vi "Get 1.3.3 Mutation Chans.vi"() -> (3 "Array":T2(array[cluster]))   [LabVIEW 2020, in "Engine Simulation Toolkit System Explorer.lvlib"]
uses:
  Engine Simulation Toolkit System Explorer.lvlib
  Shared/Channel.ctl
  Shared/Constants and GUIDs.vi
  Shared/Engine Simulation Toolkit Shared.lvlib
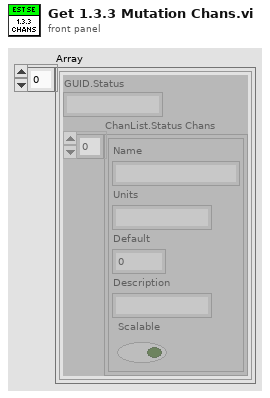
[diagram p1: front panel]
types:
  T1 = typedef "Engine Simulation Toolkit Shared.lvlib/Channel.ctl" = cluster{"Name":string, "Units":string, "Default":dbl, "Description":string, "Scalable":bool}
  T2 = cluster{"GUID.Status":string, "ChanList.Status Chans":T1[]}[]
  T3 = cluster{"GUID.APU Commands":string, "ChanList.APU Commands":T1[]}
  T4 = cluster{"GUID.APU State":string, "ChanList.APU State":T1[]}
  T5 = cluster{"GUID.Analog Replay":string, "ChanList.DataReplayVoltage":T1[]}
  T6 = cluster{"GUID.Faulting":string, "ChanList.DigPtrnFaultingIn":T1[]}
  T7 = cluster{"GUID.Faulting":string, "ChanList.DigPtrnFaultingOut":T1[]}
  T8 = cluster{"GUID.Dir Speed Sensor":string, "ChanList.DirSpeedSensor":T1[]}
  T9 = cluster{"GUID.Event Capture":string, "ChanList.EventCapture":T1[]}
  T10 = cluster{"GUID.Knock Cylinder":string, "ChanList.KnockCylinder":T1[]}
  T11 = cluster{"GUID.Knock Sensor":string, "ChanList.KnockSensor":T1[]}
  T12 = cluster{"GUID.APU State":string, "ChanList.MeasurementStatus":T1[]}
  T13 = cluster{"GUID.Analog Replay":string, "ChanList.Offset":T1[]}
  T14 = cluster{"GUID.Digital Pattern":string, "ChanList.Offset":T1[]}
  T15 = cluster{"GUID.Status":string, "ChanList.Status Chans":T1[]}
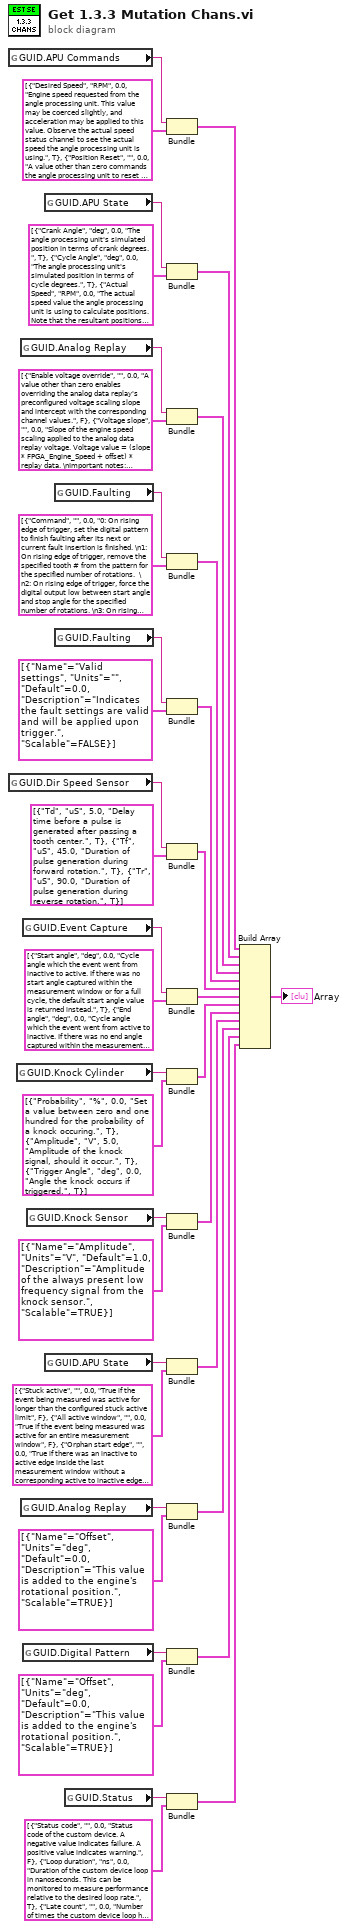
[diagram p0: block diagram]
diagram:
  n1 = global read "Constants and GUIDs.vi" "GUID.APU Commands"() -> (w33:string)
  n2 = global read "Constants and GUIDs.vi" "GUID.Dir Speed Sensor"() -> (w28:string)
  n3 = global read "Constants and GUIDs.vi" "GUID.Knock Cylinder"() -> (w26:string)
  n4 = global read "Constants and GUIDs.vi" "GUID.Analog Replay"() -> (w31:string)
  n5 = global read "Constants and GUIDs.vi" "GUID.Analog Replay"() -> (w23:string)
  n6 = global read "Constants and GUIDs.vi" "GUID.Event Capture"() -> (w27:string)
  n7 = global read "Constants and GUIDs.vi" "GUID.Digital Pattern"() -> (w22:string)
  n8 = global read "Constants and GUIDs.vi" "GUID.Knock Sensor"() -> (w25:string)
  n9 = global read "Constants and GUIDs.vi" "GUID.APU State"() -> (w32:string)
  n10 = global read "Constants and GUIDs.vi" "GUID.APU State"() -> (w24:string)
  n11 = global read "Constants and GUIDs.vi" "GUID.Faulting"() -> (w30:string)
  n12 = global read "Constants and GUIDs.vi" "GUID.Faulting"() -> (w29:string)
  n13 = global read "Constants and GUIDs.vi" "GUID.Status"() -> (w21:string)
  n14 = Bundle("GUID.APU Commands"=w33, "ChanList.APU Commands"=T1[] [{"Name"="Desired Speed", "Units"="RPM", "Default"=0.0, "Description"="Engine speed requested from the angle processing unit. This value may be coerced slightly, and acceleration may be applied to this value. Observe the actual speed status channel to see the actual speed the angle processing unit is using.", "Scalable"=TRUE}, {"Name"="Position Reset", "Units"="", "Default"=0.0, "Description"="A value other than zero commands the angle processing unit to reset to its initial position.\nWARNING: This snaps the angle processing unit position and will cause undefined behavior of output generations for a short time. For example, snapping position could cause a large instantaneous position change resulting in knock simulation generating the knock for several cylinders simultaneously. It is only recommended to reset position when the ECU under test is rebooting.\n", "Scalable"=FALSE}]) -> (w34:T3)  [unwired: 1 in]
  n15 = Bundle("GUID.APU State"=w32, "ChanList.APU State"=T1[] [{"Name"="Crank Angle", "Units"="deg", "Default"=0.0, "Description"="The angle processing unit's simulated position in terms of crank degrees.", "Scalable"=TRUE}, {"Name"="Cycle Angle", "Units"="deg", "Default"=0.0, "Description"="The angle processing unit's simulated position in terms of cycle degrees.", "Scalable"=TRUE}, {"Name"="Actual Speed", "Units"="RPM", "Default"=0.0, "Description"="The actual speed value the angle processing unit is using to calculate positions. Note that the resultant positions will slowly accumulate error as compared to the rotational speed due to numerical representation.", "Scalable"=TRUE}]) -> (w20:T4)  [unwired: 1 in]
  n16 = Bundle("GUID.Analog Replay"=w31, "ChanList.DataReplayVoltage"=T1[] [{"Name"="Enable voltage override", "Units"="", "Default"=0.0, "Description"="A value other than zero enables overriding the analog data replay's preconfigured voltage scaling slope and intercept with the corresponding channel values.", "Scalable"=FALSE}, {"Name"="Voltage slope", "Units"="", "Default"=0.0, "Description"="Slope of the engine speed scaling applied to the analog data replay voltage. Voltage value = (slope * FPGA_Engine_Speed + offset) * replay data. \nImportant notes: Replay data is always normalized to full scale range of the analog output DAC. FPGA_Engine_Speed is equal to RPM * (1/60) * (1/40M) * 2^16.", "Scalable"=TRUE}, {"Name"="Voltage intercept", "Units"="", "Default"=0.0, "Description"="Offset of the engine speed scaling applied to the analog data replay voltage. Voltage value = (slope * FPGA_Engine_Speed + offset) * replay data. \nImportant notes: Replay data is always normalized to full scale range of the analog output DAC. FPGA_Engine_Speed is equal to RPM * (1/60) * (1/40M) * 2^16.", "Scalable"=TRUE}]) -> (w19:T5)  [unwired: 1 in]
  n17 = Bundle("GUID.Faulting"=w30, "ChanList.DigPtrnFaultingIn"=T1[] [{"Name"="Command", "Units"="", "Default"=0.0, "Description"="0: On rising edge of trigger, set the digital pattern to finish faulting after its next or current fault insertion is finished. \n1: On rising edge of trigger, remove the specified tooth # from the pattern for the specified number of rotations.  \n2: On rising edge of trigger, force the digital output low between start angle and stop angle for the specified number of rotations. \n3: On rising edge of trigger, force the digital output high between start angle and stop angle for the specified number of rotations.", "Scalable"=FALSE}, {"Name"="Trigger", "Units"="", "Default"=0.0, "Description"="Ignored if valid settings is false.", "Scalable"=FALSE}, {"Name"="Rotations", "Units"="", "Default"=0.0, "Description"="Up to 16. 0 means indefinitely until faulting is commanded to finish.", "Scalable"=FALSE}, {"Name"="Start angle", "Units"="deg", "Default"=0.0, "Description"="Rotational position to begin faulting.", "Scalable"=TRUE}, {"Name"="Stop angle", "Units"="deg", "Default"=0.0, "Description"="Rotational position to end faulting.", "Scalable"=TRUE}, {"Name"="Tooth to remove", "Units"="", "Default"=0.0, "Description"="Tooth number of the pattern to remove during faulting. Teeth are 1 indexed from the begining of the rotation (crank or cycle) to the end.", "Scalable"=TRUE}]) -> (w18:T6)  [unwired: 1 in]
  n18 = Bundle("GUID.Faulting"=w29, "ChanList.DigPtrnFaultingOut"=T1[] [{"Name"="Valid settings", "Units"="", "Default"=0.0, "Description"="Indicates the fault settings are valid and will be applied upon trigger.", "Scalable"=FALSE}]) -> (w17:T7)  [unwired: 1 in]
  n19 = Bundle("GUID.Dir Speed Sensor"=w28, "ChanList.DirSpeedSensor"=T1[] [{"Name"="Td", "Units"="uS", "Default"=5.0, "Description"="Delay time before a pulse is generated after passing a tooth center.", "Scalable"=TRUE}, {"Name"="Tf", "Units"="uS", "Default"=45.0, "Description"="Duration of pulse generation during forward rotation.", "Scalable"=TRUE}, {"Name"="Tr", "Units"="uS", "Default"=90.0, "Description"="Duration of pulse generation during reverse rotation.", "Scalable"=TRUE}]) -> (w16:T8)  [unwired: 1 in]
  n20 = Bundle("GUID.Event Capture"=w27, "ChanList.EventCapture"=T1[] [{"Name"="Start angle", "Units"="deg", "Default"=0.0, "Description"="Cycle angle which the event went from inactive to active. If there was no start angle captured within the measurement window or for a full cycle, the default start angle value is returned instead.", "Scalable"=TRUE}, {"Name"="End angle", "Units"="deg", "Default"=0.0, "Description"="Cycle angle which the event went from active to inactive. If there was no end angle captured within the measurement window or for a full cycle, the default end angle value is returned instead.", "Scalable"=TRUE}, {"Name"="Duration", "Units"="ms", "Default"=0.0, "Description"="Duration of event active time within the measurement window.", "Scalable"=TRUE}]) -> (w15:T9)  [unwired: 1 in]
  n21 = Bundle("GUID.Knock Cylinder"=w26, "ChanList.KnockCylinder"=T1[] [{"Name"="Probability", "Units"="%", "Default"=0.0, "Description"="Set a value between zero and one hundred for the probability of a knock occuring.", "Scalable"=TRUE}, {"Name"="Amplitude", "Units"="V", "Default"=5.0, "Description"="Amplitude of the knock signal, should it occur.", "Scalable"=TRUE}, {"Name"="Trigger Angle", "Units"="deg", "Default"=0.0, "Description"="Angle the knock occurs if triggered.", "Scalable"=TRUE}]) -> (w14:T10)  [unwired: 1 in]
  n22 = Bundle("GUID.Knock Sensor"=w25, "ChanList.KnockSensor"=T1[] [{"Name"="Amplitude", "Units"="V", "Default"=1.0, "Description"="Amplitude of the always present low frequency signal from the knock sensor.", "Scalable"=TRUE}]) -> (w13:T11)  [unwired: 1 in]
  n23 = Bundle("GUID.APU State"=w24, "ChanList.MeasurementStatus"=T1[] [{"Name"="Stuck active", "Units"="", "Default"=0.0, "Description"="True if the event being measured was active for longer than the configured stuck active limit", "Scalable"=FALSE}, {"Name"="All active window", "Units"="", "Default"=0.0, "Description"="True if the event being measured was active for an entire measurement window", "Scalable"=FALSE}, {"Name"="Orphan start edge", "Units"="", "Default"=0.0, "Description"="True if there was an inactive to active edge inside the last measurement window without a corresponding active to inactive edge.", "Scalable"=FALSE}, {"Name"="Orphan end edge", "Units"="", "Default"=0.0, "Description"="True if there was an active to inactive edge inside the last measurement window without a corresponding inactive to active edge.", "Scalable"=FALSE}]) -> (w12:T12)  [unwired: 1 in]
  n24 = Bundle("GUID.Analog Replay"=w23, "ChanList.Offset"=T1[] [{"Name"="Offset", "Units"="deg", "Default"=0.0, "Description"="This value is added to the engine's rotational position.", "Scalable"=TRUE}]) -> (w11:T13)  [unwired: 1 in]
  n25 = Bundle("GUID.Digital Pattern"=w22, "ChanList.Offset"=T1[] [{"Name"="Offset", "Units"="deg", "Default"=0.0, "Description"="This value is added to the engine's rotational position.", "Scalable"=TRUE}]) -> (w10:T14)  [unwired: 1 in]
  n26 = Bundle("GUID.Status"=w21, "ChanList.Status Chans"=T1[] [{"Name"="Status code", "Units"="", "Default"=0.0, "Description"="Status code of the custom device. A negative value indicates failure. A positive value indicates warning.", "Scalable"=FALSE}, {"Name"="Loop duration", "Units"="ns", "Default"=0.0, "Description"="Duration of the custom device loop in nanoseconds. This can be monitored to measure performance relative to the desired loop rate.", "Scalable"=TRUE}, {"Name"="Late count", "Units"="", "Default"=0.0, "Description"="Number of times the custom device loop has gone late.", "Scalable"=FALSE}]) -> (w9:T15)  [unwired: 1 in]
  n27 = Build Array(w34, w20, w19, w18, w17, w16, w15, w14, w13, w12, w11, w10, w9) -> (→"Array":T2)
